vi "App - analyze RUS V6.vi"() -> ()   [LabVIEW 2018] (continued)
{"temperature"=14.948, "lorentzian"={"A (VHz)"=0.0, "f (Hz)"=0.0, "G (Hz)"=0.0, "phi(rad)"=0.0, "Q"=0.0, "Norm  Ampl"=0.0, "bg (V)"=0.0+0.0i, "4corners"={"z (-pi/2)"=0.0+0.0i, "z(inf)"=0.0+0.0i, "z (pi/2)"=0.0+0.0i, "z center"=0.0+0.0i, "z(0)"=0.0+0.0i, "radius"=0.0}}, "timestamp(min)"=2008.2666666656733, "timestamp"=timestamp(3493848317 s since 1904-01-01), "Magn Field(T)"=0.0}, {"temperature"=14.938, "lorentzian"={"A (VHz)"=0.0, "f (Hz)"=0.0, "G (Hz)"=0.0, "phi(rad)"=0.0, "Q"=0.0, "Norm  Ampl"=0.0, "bg (V)"=0.0+0.0i, "4corners"={"z (-pi/2)"=0.0+0.0i, "z(inf)"=0.0+0.0i, "z (pi/2)"=0.0+0.0i, "z center"=0.0+0.0i, "z(0)"=0.0+0.0i, "radius"=0.0}}, "timestamp(min)"=2009.6000000014901, "timestamp"=timestamp(3493848397 s since 1904-01-01), "Magn Field(T)"=0.0}, {"temperature"=14.942, "lorentzian"={"A (VHz)"=0.0, "f (Hz)"=0.0, "G (Hz)"=0.0, "phi(rad)"=0.0, "Q"=0.0, "Norm  Ampl"=0.0, "bg (V)"=0.0+0.0i, "4corners"={"z (-pi/2)"=0.0+0.0i, "z(inf)"=0.0+0.0i, "z (pi/2)"=0.0+0.0i, "z center"=0.0+0.0i, "z(0)"=0.0+0.0i, "radius"=0.0}}, "timestamp(min)"=2010.9166666641831, "timestamp"=timestamp(3493848476 s since 1904-01-01), "Magn Field(T)"=0.0}, {"temperature"=14.929, "lorentzian"={"A (VHz)"=0.0, "f (Hz)"=0.0, "G (Hz)"=0.0, "phi(rad)"=0.0, "Q"=0.0, "Norm  Ampl"=0.0, "bg (V)"=0.0+0.0i, "4corners"={"z (-pi/2)"=0.0+0.0i, "z(inf)"=0.0+0.0i, "z (pi/2)"=0.0+0.0i, "z center"=0.0+0.0i, "z(0)"=0.0+0.0i, "radius"=0.0}}, "timestamp(min)"=2012.2333333343267, "timestamp"=timestamp(3493848555 s since 1904-01-01), "Magn Field(T)"=0.0}, {"temperature"=14.927, "lorentzian"={"A (VHz)"=0.0, "f (Hz)"=0.0, "G (Hz)"=0.0, "phi(rad)"=0.0, "Q"=0.0, "Norm  Ampl"=0.0, "bg (V)"=0.0+0.0i, "4corners"={"z (-pi/2)"=0.0+0.0i, "z(inf)"=0.0+0.0i, "z (pi/2)"=0.0+0.0i, "z center"=0.0+0.0i, "z(0)"=0.0+0.0i, "radius"=0.0}}, "timestamp(min)"=2013.5666666701436, "timestamp"=timestamp(3493848635 s since 1904-01-01), "Magn Field(T)"=0.0}, {"temperature"=14.922, "lorentzian"={"A (VHz)"=0.0, "f (Hz)"=0.0, "G (Hz)"=0.0, "phi(rad)"=0.0, "Q"=0.0, "Norm  Ampl"=0.0, "bg (V)"=0.0+0.0i, "4corners"={"z (-pi/2)"=0.0+0.0i, "z(inf)"=0.0+0.0i, "z (pi/2)"=0.0+0.0i, "z center"=0.0+0.0i, "z(0)"=0.0+0.0i, "radius"=0.0}}, "timestamp(min)"=2014.8833333328366, "timestamp"=timestamp(3493848714 s since 1904-01-01), "Magn Field(T)"=0.0}, {"temperature"=14.929, "lorentzian"={"A (VHz)"=0.0, "f (Hz)"=0.0, "G (Hz)"=0.0, "phi(rad)"=0.0, "Q"=0.0, "Norm  Ampl"=0.0, "bg (V)"=0.0+0.0i, "4corners"={"z (-pi/2)"=0.0+0.0i, "z(inf)"=0.0+0.0i, "z (pi/2)"=0.0+0.0i, "z center"=0.0+0.0i, "z(0)"=0.0+0.0i, "radius"=0.0}}, "timestamp(min)"=2016.2166666686535, "timestamp"=timestamp(3493848794 s since 1904-01-01), "Magn Field(T)"=0.0}, {"temperature"=14.927, "lorentzian"={"A (VHz)"=0.0, "f (Hz)"=0.0, "G (Hz)"=0.0, "phi(rad)"=0.0, "Q"=0.0, "Norm  Ampl"=0.0, "bg (V)"=0.0+0.0i, "4corners"={"z (-pi/2)"=0.0+0.0i, "z(inf)"=0.0+0.0i, "z (pi/2)"=0.0+0.0i, "z center"=0.0+0.0i, "z(0)"=0.0+0.0i, "radius"=0.0}}, "timestamp(min)"=2017.5333333313465, "timestamp"=timestamp(3493848873 s since 1904-01-01), "Magn Field(T)"=0.0}, {"temperature"=14.926, "lorentzian"={"A (VHz)"=0.0, "f (Hz)"=0.0, "G (Hz)"=0.0, "phi(rad)"=0.0, "Q"=0.0, "Norm  Ampl"=0.0, "bg (V)"=0.0+0.0i, "4corners"={"z (-pi/2)"=0.0+0.0i, "z(inf)"=0.0+0.0i, "z (pi/2)"=0.0+0.0i, "z center"=0.0+0.0i, "z(0)"=0.0+0.0i, "radius"=0.0}}, "timestamp(min)"=2018.8500000014901, "timestamp"=timestamp(3493848952 s since 1904-01-01), "Magn Field(T)"=0.0}, {"temperature"=14.912, "lorentzian"={"A (VHz)"=0.0, "f (Hz)"=0.0, "G (Hz)"=0.0, "phi(rad)"=0.0, "Q"=0.0, "Norm  Ampl"=0.0, "bg (V)"=0.0+0.0i, "4corners"={"z (-pi/2)"=0.0+0.0i, "z(inf)"=0.0+0.0i, "z (pi/2)"=0.0+0.0i, "z center"=0.0+0.0i, "z(0)"=0.0+0.0i, "radius"=0.0}}, "timestamp(min)"=2020.183333337307, "timestamp"=timestamp(3493849032 s since 1904-01-01), "Magn Field(T)"=0.0}, {"temperature"=14.915, "lorentzian"={"A (VHz)"=0.0, "f (Hz)"=0.0, "G (Hz)"=0.0, "phi(rad)"=0.0, "Q"=0.0, "Norm  Ampl"=0.0, "bg (V)"=0.0+0.0i, "4corners"={"z (-pi/2)"=0.0+0.0i, "z(inf)"=0.0+0.0i, "z (pi/2)"=0.0+0.0i, "z center"=0.0+0.0i, "z(0)"=0.0+0.0i, "radius"=0.0}}, "timestamp(min)"=2021.5, "timestamp"=timestamp(3493849111 s since 1904-01-01), "Magn Field(T)"=0.0}, {"temperature"=14.912, "lorentzian"={"A (VHz)"=0.0, "f (Hz)"=0.0, "G (Hz)"=0.0, "phi(rad)"=0.0, "Q"=0.0, "Norm  Ampl"=0.0, "bg (V)"=0.0+0.0i, "4corners"={"z (-pi/2)"=0.0+0.0i, "z(inf)"=0.0+0.0i, "z (pi/2)"=0.0+0.0i, "z center"=0.0+0.0i, "z(0)"=0.0+0.0i, "radius"=0.0}}, "timestamp(min)"=2022.8166666701436, "timestamp"=timestamp(3493849190 s since 1904-01-01), "Magn Field(T)"=0.0}, {"temperature"=14.91, "lorentzian"={"A (VHz)"=0.0, "f (Hz)"=0.0, "G (Hz)"=0.0, "phi(rad)"=0.0, "Q"=0.0, "Norm  Ampl"=0.0, "bg (V)"=0.0+0.0i, "4corners"={"z (-pi/2)"=0.0+0.0i, "z(inf)"=0.0+0.0i, "z (pi/2)"=0.0+0.0i, "z center"=0.0+0.0i, "z(0)"=0.0+0.0i, "radius"=0.0}}, "timestamp(min)"=2024.1499999985099, "timestamp"=timestamp(3493849270 s since 1904-01-01), "Magn Field(T)"=0.0}, {"temperature"=14.907, "lorentzian"={"A (VHz)"=0.0, "f (Hz)"=0.0, "G (Hz)"=0.0, "phi(rad)"=0.0, "Q"=0.0, "Norm  Ampl"=0.0, "bg (V)"=0.0+0.0i, "4corners"={"z (-pi/2)"=0.0+0.0i, "z(inf)"=0.0+0.0i, "z (pi/2)"=0.0+0.0i, "z center"=0.0+0.0i, "z(0)"=0.0+0.0i, "radius"=0.0}}, "timestamp(min)"=2025.4666666686535, "timestamp"=timestamp(3493849349 s since 1904-01-01), "Magn Field(T)"=0.0}, {"temperature"=14.908, "lorentzian"={"A (VHz)"=0.0, "f (Hz)"=0.0, "G (Hz)"=0.0, "phi(rad)"=0.0, "Q"=0.0, "Norm  Ampl"=0.0, "bg (V)"=0.0+0.0i, "4corners"={"z (-pi/2)"=0.0+0.0i, "z(inf)"=0.0+0.0i, "z (pi/2)"=0.0+0.0i, "z center"=0.0+0.0i, "z(0)"=0.0+0.0i, "radius"=0.0}}, "timestamp(min)"=2026.8000000044703, "timestamp"=timestamp(3493849429 s since 1904-01-01), "Magn Field(T)"=0.0}, {"temperature"=14.9, "lorentzian"={"A (VHz)"=0.0, "f (Hz)"=0.0, "G (Hz)"=0.0, "phi(rad)"=0.0, "Q"=0.0, "Norm  Ampl"=0.0, "bg (V)"=0.0+0.0i, "4corners"={"z (-pi/2)"=0.0+0.0i, "z(inf)"=0.0+0.0i, "z (pi/2)"=0.0+0.0i, "z center"=0.0+0.0i, "z(0)"=0.0+0.0i, "radius"=0.0}}, "timestamp(min)"=2028.1166666671634, "timestamp"=timestamp(3493849508 s since 1904-01-01), "Magn Field(T)"=0.0}, {"temperature"=14.9, "lorentzian"={"A (VHz)"=0.0, "f (Hz)"=0.0, "G (Hz)"=0.0, "phi(rad)"=0.0, "Q"=0.0, "Norm  Ampl"=0.0, "bg (V)"=0.0+0.0i, "4corners"={"z (-pi/2)"=0.0+0.0i, "z(inf)"=0.0+0.0i, "z (pi/2)"=0.0+0.0i, "z center"=0.0+0.0i, "z(0)"=0.0+0.0i, "radius"=0.0}}, "timestamp(min)"=2029.433333337307, "timestamp"=timestamp(3493849587 s since 1904-01-01), "Magn Field(T)"=0.0}, {"temperature"=14.895, "lorentzian"={"A (VHz)"=0.0, "f (Hz)"=0.0, "G (Hz)"=0.0, "phi(rad)"=0.0, "Q"=0.0, "Norm  Ampl"=0.0, "bg (V)"=0.0+0.0i, "4corners"={"z (-pi/2)"=0.0+0.0i, "z(inf)"=0.0+0.0i, "z (pi/2)"=0.0+0.0i, "z center"=0.0+0.0i, "z(0)"=0.0+0.0i, "radius"=0.0}}, "timestamp(min)"=2030.7666666656733, "timestamp"=timestamp(3493849667 s since 1904-01-01), "Magn Field(T)"=0.0}, {"temperature"=14.89, "lorentzian"={"A (VHz)"=0.0, "f (Hz)"=0.0, "G (Hz)"=0.0, "phi(rad)"=0.0, "Q"=0.0, "Norm  Ampl"=0.0, "bg (V)"=0.0+0.0i, "4corners"={"z (-pi/2)"=0.0+0.0i, "z(inf)"=0.0+0.0i, "z (pi/2)"=0.0+0.0i, "z center"=0.0+0.0i, "z(0)"=0.0+0.0i, "radius"=0.0}}, "timestamp(min)"=2032.0833333358169, "timestamp"=timestamp(3493849746 s since 1904-01-01), "Magn Field(T)"=0.0}, {"temperature"=14.886, "lorentzian"={"A (VHz)"=0.0, "f (Hz)"=0.0, "G (Hz)"=0.0, "phi(rad)"=0.0, "Q"=0.0, "Norm  Ampl"=0.0, "bg (V)"=0.0+0.0i, "4corners"={"z (-pi/2)"=0.0+0.0i, "z(inf)"=0.0+0.0i, "z (pi/2)"=0.0+0.0i, "z center"=0.0+0.0i, "z(0)"=0.0+0.0i, "radius"=0.0}}, "timestamp(min)"=2033.4166666641831, "timestamp"=timestamp(3493849826 s since 1904-01-01), "Magn Field(T)"=0.0}, {"temperature"=14.883, "lorentzian"={"A (VHz)"=0.0, "f (Hz)"=0.0, "G (Hz)"=0.0, "phi(rad)"=0.0, "Q"=0.0, "Norm  Ampl"=0.0, "bg (V)"=0.0+0.0i, "4corners"={"z (-pi/2)"=0.0+0.0i, "z(inf)"=0.0+0.0i, "z (pi/2)"=0.0+0.0i, "z center"=0.0+0.0i, "z(0)"=0.0+0.0i, "radius"=0.0}}, "timestamp(min)"=2034.7333333343267, "timestamp"=timestamp(3493849905 s since 1904-01-01), "Magn Field(T)"=0.0}, {"temperature"=14.876, "lorentzian"={"A (VHz)"=0.0, "f (Hz)"=0.0, "G (Hz)"=0.0, "phi(rad)"=0.0, "Q"=0.0, "Norm  Ampl"=0.0, "bg (V)"=0.0+0.0i, "4corners"={"z (-pi/2)"=0.0+0.0i, "z(inf)"=0.0+0.0i, "z (pi/2)"=0.0+0.0i, "z center"=0.0+0.0i, "z(0)"=0.0+0.0i, "radius"=0.0}}, "timestamp(min)"=2036.0500000044703, "timestamp"=timestamp(3493849984 s since 1904-01-01), "Magn Field(T)"=0.0}, {"temperature"=14.875, "lorentzian"={"A (VHz)"=0.0, "f (Hz)"=0.0, "G (Hz)"=0.0, "phi(rad)"=0.0, "Q"=0.0, "Norm  Ampl"=0.0, "bg (V)"=0.0+0.0i, "4corners"={"z (-pi/2)"=0.0+0.0i, "z(inf)"=0.0+0.0i, "z (pi/2)"=0.0+0.0i, "z center"=0.0+0.0i, "z(0)"=0.0+0.0i, "radius"=0.0}}, "timestamp(min)"=2037.3833333328366, "timestamp"=timestamp(3493850064 s since 1904-01-01), "Magn Field(T)"=0.0}, {"temperature"=14.872, "lorentzian"={"A (VHz)"=0.0, "f (Hz)"=0.0, "G (Hz)"=0.0, "phi(rad)"=0.0, "Q"=0.0, "Norm  Ampl"=0.0, "bg (V)"=0.0+0.0i, "4corners"={"z (-pi/2)"=0.0+0.0i, "z(inf)"=0.0+0.0i, "z (pi/2)"=0.0+0.0i, "z center"=0.0+0.0i, "z(0)"=0.0+0.0i, "radius"=0.0}}, "timestamp(min)"=2038.7000000029802, "timestamp"=timestamp(3493850143 s since 1904-01-01), "Magn Field(T)"=0.0}, {"temperature"=14.874, "lorentzian"={"A (VHz)"=0.0, "f (Hz)"=0.0, "G (Hz)"=0.0, "phi(rad)"=0.0, "Q"=0.0, "Norm  Ampl"=0.0, "bg (V)"=0.0+0.0i, "4corners"={"z (-pi/2)"=0.0+0.0i, "z(inf)"=0.0+0.0i, "z (pi/2)"=0.0+0.0i, "z center"=0.0+0.0i, "z(0)"=0.0+0.0i, "radius"=0.0}}, "timestamp(min)"=2040.0166666656733, "timestamp"=timestamp(3493850222 s since 1904-01-01), "Magn Field(T)"=0.0}, {"temperature"=14.877, "lorentzian"={"A (VHz)"=0.0, "f (Hz)"=0.0, "G (Hz)"=0.0, "phi(rad)"=0.0, "Q"=0.0, "Norm  Ampl"=0.0, "bg (V)"=0.0+0.0i, "4corners"={"z (-pi/2)"=0.0+0.0i, "z(inf)"=0.0+0.0i, "z (pi/2)"=0.0+0.0i, "z center"=0.0+0.0i, "z(0)"=0.0+0.0i, "radius"=0.0}}, "timestamp(min)"=2041.3500000014901, "timestamp"=timestamp(3493850302 s since 1904-01-01), "Magn Field(T)"=0.0}, {"temperature"=14.872, "lorentzian"={"A (VHz)"=0.0, "f (Hz)"=0.0, "G (Hz)"=0.0, "phi(rad)"=0.0, "Q"=0.0, "Norm  Ampl"=0.0, "bg (V)"=0.0+0.0i, "4corners"={"z (-pi/2)"=0.0+0.0i, "z(inf)"=0.0+0.0i, "z (pi/2)"=0.0+0.0i, "z center"=0.0+0.0i, "z(0)"=0.0+0.0i, "radius"=0.0}}, "timestamp(min)"=2042.6666666641831, "timestamp"=timestamp(3493850381 s since 1904-01-01), "Magn Field(T)"=0.0}, {"temperature"=14.873, "lorentzian"={"A (VHz)"=0.0, "f (Hz)"=0.0, "G (Hz)"=0.0, "phi(rad)"=0.0, "Q"=0.0, "Norm  Ampl"=0.0, "bg (V)"=0.0+0.0i, "4corners"={"z (-pi/2)"=0.0+0.0i, "z(inf)"=0.0+0.0i, "z (pi/2)"=0.0+0.0i, "z center"=0.0+0.0i, "z(0)"=0.0+0.0i, "radius"=0.0}}, "timestamp(min)"=2044.0, "timestamp"=timestamp(3493850461 s since 1904-01-01), "Magn Field(T)"=0.0}, {"temperature"=14.873, "lorentzian"={"A (VHz)"=0.0, "f (Hz)"=0.0, "G (Hz)"=0.0, "phi(rad)"=0.0, "Q"=0.0, "Norm  Ampl"=0.0, "bg (V)"=0.0+0.0i, "4corners"={"z (-pi/2)"=0.0+0.0i, "z(inf)"=0.0+0.0i, "z (pi/2)"=0.0+0.0i, "z center"=0.0+0.0i, "z(0)"=0.0+0.0i, "radius"=0.0}}, "timestamp(min)"=2045.3166666701436, "timestamp"=timestamp(3493850540 s since 1904-01-01), "Magn Field(T)"=0.0}, {"temperature"=14.868, "lorentzian"={"A (VHz)"=0.0, "f (Hz)"=0.0, "G (Hz)"=0.0, "phi(rad)"=0.0, "Q"=0.0, "Norm  Ampl"=0.0, "bg (V)"=0.0+0.0i, "4corners"={"z (-pi/2)"=0.0+0.0i, "z(inf)"=0.0+0.0i, "z (pi/2)"=0.0+0.0i, "z center"=0.0+0.0i, "z(0)"=0.0+0.0i, "radius"=0.0}}, "timestamp(min)"=2046.6333333328366, "timestamp"=timestamp(3493850619 s since 1904-01-01), "Magn Field(T)"=0.0}, {"temperature"=14.859, "lorentzian"={"A (VHz)"=0.0, "f (Hz)"=0.0, "G (Hz)"=0.0, "phi(rad)"=0.0, "Q"=0.0, "Norm  Ampl"=0.0, "bg (V)"=0.0+0.0i, "4corners"={"z (-pi/2)"=0.0+0.0i, "z(inf)"=0.0+0.0i, "z (pi/2)"=0.0+0.0i, "z center"=0.0+0.0i, "z(0)"=0.0+0.0i, "radius"=0.0}}, "timestamp(min)"=2047.9666666686535, "timestamp"=timestamp(3493850699 s since 1904-01-01), "Magn Field(T)"=0.0}, {"temperature"=14.866, "lorentzian"={"A (VHz)"=0.0, "f (Hz)"=0.0, "G (Hz)"=0.0, "phi(rad)"=0.0, "Q"=0.0, "Norm  Ampl"=0.0, "bg (V)"=0.0+0.0i, "4corners"={"z (-pi/2)"=0.0+0.0i, "z(inf)"=0.0+0.0i, "z (pi/2)"=0.0+0.0i, "z center"=0.0+0.0i, "z(0)"=0.0+0.0i, "radius"=0.0}}, "timestamp(min)"=2049.2833333313465, "timestamp"=timestamp(3493850778 s since 1904-01-01), "Magn Field(T)"=0.0}, {"temperature"=14.858, "lorentzian"={"A (VHz)"=0.0, "f (Hz)"=0.0, "G (Hz)"=0.0, "phi(rad)"=0.0, "Q"=0.0, "Norm  Ampl"=0.0, "bg (V)"=0.0+0.0i, "4corners"={"z (-pi/2)"=0.0+0.0i, "z(inf)"=0.0+0.0i, "z (pi/2)"=0.0+0.0i, "z center"=0.0+0.0i, "z(0)"=0.0+0.0i, "radius"=0.0}}, "timestamp(min)"=2050.60000000149, "timestamp"=timestamp(3493850857 s since 1904-01-01), "Magn Field(T)"=0.0}, {"temperature"=14.86, "lorentzian"={"A (VHz)"=0.0, "f (Hz)"=0.0, "G (Hz)"=0.0, "phi(rad)"=0.0, "Q"=0.0, "Norm  Ampl"=0.0, "bg (V)"=0.0+0.0i, "4corners"={"z (-pi/2)"=0.0+0.0i, "z(inf)"=0.0+0.0i, "z (pi/2)"=0.0+0.0i, "z center"=0.0+0.0i, "z(0)"=0.0+0.0i, "radius"=0.0}}, "timestamp(min)"=2051.933333337307, "timestamp"=timestamp(3493850937 s since 1904-01-01), "Magn Field(T)"=0.0}, {"temperature"=14.866, "lorentzian"={"A (VHz)"=0.0, "f (Hz)"=0.0, "G (Hz)"=0.0, "phi(rad)"=0.0, "Q"=0.0, "Norm  Ampl"=0.0, "bg (V)"=0.0+0.0i, "4corners"={"z (-pi/2)"=0.0+0.0i, "z(inf)"=0.0+0.0i, "z (pi/2)"=0.0+0.0i, "z center"=0.0+0.0i, "z(0)"=0.0+0.0i, "radius"=0.0}}, "timestamp(min)"=2053.25, "timestamp"=timestamp(3493851016 s since 1904-01-01), "Magn Field(T)"=0.0}, {"temperature"=14.857, "lorentzian"={"A (VHz)"=0.0, "f (Hz)"=0.0, "G (Hz)"=0.0, "phi(rad)"=0.0, "Q"=0.0, "Norm  Ampl"=0.0, "bg (V)"=0.0+0.0i, "4corners"={"z (-pi/2)"=0.0+0.0i, "z(inf)"=0.0+0.0i, "z (pi/2)"=0.0+0.0i, "z center"=0.0+0.0i, "z(0)"=0.0+0.0i, "radius"=0.0}}, "timestamp(min)"=2054.583333335817, "timestamp"=timestamp(3493851096 s since 1904-01-01), "Magn Field(T)"=0.0}, {"temperature"=14.853, "lorentzian"={"A (VHz)"=0.0, "f (Hz)"=0.0, "G (Hz)"=0.0, "phi(rad)"=0.0, "Q"=0.0, "Norm  Ampl"=0.0, "bg (V)"=0.0+0.0i, "4corners"={"z (-pi/2)"=0.0+0.0i, "z(inf)"=0.0+0.0i, "z (pi/2)"=0.0+0.0i, "z center"=0.0+0.0i, "z(0)"=0.0+0.0i, "radius"=0.0}}, "timestamp(min)"=2055.89999999851, "timestamp"=timestamp(3493851175 s since 1904-01-01), "Magn Field(T)"=0.0}, {"temperature"=14.852, "lorentzian"={"A (VHz)"=0.0, "f (Hz)"=0.0, "G (Hz)"=0.0, "phi(rad)"=0.0, "Q"=0.0, "Norm  Ampl"=0.0, "bg (V)"=0.0+0.0i, "4corners"={"z (-pi/2)"=0.0+0.0i, "z(inf)"=0.0+0.0i, "z (pi/2)"=0.0+0.0i, "z center"=0.0+0.0i, "z(0)"=0.0+0.0i, "radius"=0.0}}, "timestamp(min)"=2057.2166666686535, "timestamp"=timestamp(3493851254 s since 1904-01-01), "Magn Field(T)"=0.0}, {"temperature"=14.844, "lorentzian"={"A (VHz)"=0.0, "f (Hz)"=0.0, "G (Hz)"=0.0, "phi(rad)"=0.0, "Q"=0.0, "Norm  Ampl"=0.0, "bg (V)"=0.0+0.0i, "4corners"={"z (-pi/2)"=0.0+0.0i, "z(inf)"=0.0+0.0i, "z (pi/2)"=0.0+0.0i, "z center"=0.0+0.0i, "z(0)"=0.0+0.0i, "radius"=0.0}}, "timestamp(min)"=2058.5500000044703, "timestamp"=timestamp(3493851334 s since 1904-01-01), "Magn Field(T)"=0.0}, {"temperature"=14.841, "lorentzian"={"A (VHz)"=0.0, "f (Hz)"=0.0, "G (Hz)"=0.0, "phi(rad)"=0.0, "Q"=0.0, "Norm  Ampl"=0.0, "bg (V)"=0.0+0.0i, "4corners"={"z (-pi/2)"=0.0+0.0i, "z(inf)"=0.0+0.0i, "z (pi/2)"=0.0+0.0i, "z center"=0.0+0.0i, "z(0)"=0.0+0.0i, "radius"=0.0}}, "timestamp(min)"=2059.8666666671634, "timestamp"=timestamp(3493851413 s since 1904-01-01), "Magn Field(T)"=0.0}, {"temperature"=14.835, "lorentzian"={"A (VHz)"=0.0, "f (Hz)"=0.0, "G (Hz)"=0.0, "phi(rad)"=0.0, "Q"=0.0, "Norm  Ampl"=0.0, "bg (V)"=0.0+0.0i, "4corners"={"z (-pi/2)"=0.0+0.0i, "z(inf)"=0.0+0.0i, "z (pi/2)"=0.0+0.0i, "z center"=0.0+0.0i, "z(0)"=0.0+0.0i, "radius"=0.0}}, "timestamp(min)"=2061.183333337307, "timestamp"=timestamp(3493851492 s since 1904-01-01), "Magn Field(T)"=0.0}, {"temperature"=14.822, "lorentzian"={"A (VHz)"=0.0, "f (Hz)"=0.0, "G (Hz)"=0.0, "phi(rad)"=0.0, "Q"=0.0, "Norm  Ampl"=0.0, "bg (V)"=0.0+0.0i, "4corners"={"z (-pi/2)"=0.0+0.0i, "z(inf)"=0.0+0.0i, "z (pi/2)"=0.0+0.0i, "z center"=0.0+0.0i, "z(0)"=0.0+0.0i, "radius"=0.0}}, "timestamp(min)"=2062.5166666656733, "timestamp"=timestamp(3493851572 s since 1904-01-01), "Magn Field(T)"=0.0}, {"temperature"=14.821, "lorentzian"={"A (VHz)"=0.0, "f (Hz)"=0.0, "G (Hz)"=0.0, "phi(rad)"=0.0, "Q"=0.0, "Norm  Ampl"=0.0, "bg (V)"=0.0+0.0i, "4corners"={"z (-pi/2)"=0.0+0.0i, "z(inf)"=0.0+0.0i, "z (pi/2)"=0.0+0.0i, "z center"=0.0+0.0i, "z(0)"=0.0+0.0i, "radius"=0.0}}, "timestamp(min)"=2063.833333335817, "timestamp"=timestamp(3493851651 s since 1904-01-01), "Magn Field(T)"=0.0}, {"temperature"=14.824, "lorentzian"={"A (VHz)"=0.0, "f (Hz)"=0.0, "G (Hz)"=0.0, "phi(rad)"=0.0, "Q"=0.0, "Norm  Ampl"=0.0, "bg (V)"=0.0+0.0i, "4corners"={"z (-pi/2)"=0.0+0.0i, "z(inf)"=0.0+0.0i, "z (pi/2)"=0.0+0.0i, "z center"=0.0+0.0i, "z(0)"=0.0+0.0i, "radius"=0.0}}, "timestamp(min)"=2065.166666664183, "timestamp"=timestamp(3493851731 s since 1904-01-01), "Magn Field(T)"=0.0}, {"temperature"=14.817, "lorentzian"={"A (VHz)"=0.0, "f (Hz)"=0.0, "G (Hz)"=0.0, "phi(rad)"=0.0, "Q"=0.0, "Norm  Ampl"=0.0, "bg (V)"=0.0+0.0i, "4corners"={"z (-pi/2)"=0.0+0.0i, "z(inf)"=0.0+0.0i, "z (pi/2)"=0.0+0.0i, "z center"=0.0+0.0i, "z(0)"=0.0+0.0i, "radius"=0.0}}, "timestamp(min)"=2066.4833333343267, "timestamp"=timestamp(3493851810 s since 1904-01-01), "Magn Field(T)"=0.0}, {"temperature"=14.811, "lorentzian"={"A (VHz)"=0.0, "f (Hz)"=0.0, "G (Hz)"=0.0, "phi(rad)"=0.0, "Q"=0.0, "Norm  Ampl"=0.0, "bg (V)"=0.0+0.0i, "4corners"={"z (-pi/2)"=0.0+0.0i, "z(inf)"=0.0+0.0i, "z (pi/2)"=0.0+0.0i, "z center"=0.0+0.0i, "z(0)"=0.0+0.0i, "radius"=0.0}}, "timestamp(min)"=2067.8000000044703, "timestamp"=timestamp(3493851889 s since 1904-01-01), "Magn Field(T)"=0.0}, {"temperature"=14.805, "lorentzian"={"A (VHz)"=0.0, "f (Hz)"=0.0, "G (Hz)"=0.0, "phi(rad)"=0.0, "Q"=0.0, "Norm  Ampl"=0.0, "bg (V)"=0.0+0.0i, "4corners"={"z (-pi/2)"=0.0+0.0i, "z(inf)"=0.0+0.0i, "z (pi/2)"=0.0+0.0i, "z center"=0.0+0.0i, "z(0)"=0.0+0.0i, "radius"=0.0}}, "timestamp(min)"=2069.1333333328366, "timestamp"=timestamp(3493851969 s since 1904-01-01), "Magn Field(T)"=0.0}, {"temperature"=14.791, "lorentzian"={"A (VHz)"=0.0, "f (Hz)"=0.0, "G (Hz)"=0.0, "phi(rad)"=0.0, "Q"=0.0, "Norm  Ampl"=0.0, "bg (V)"=0.0+0.0i, "4corners"={"z (-pi/2)"=0.0+0.0i, "z(inf)"=0.0+0.0i, "z (pi/2)"=0.0+0.0i, "z center"=0.0+0.0i, "z(0)"=0.0+0.0i, "radius"=0.0}}, "timestamp(min)"=2070.4500000029802, "timestamp"=timestamp(3493852048 s since 1904-01-01), "Magn Field(T)"=0.0}, {"temperature"=14.787, "lorentzian"={"A (VHz)"=0.0, "f (Hz)"=0.0, "G (Hz)"=0.0, "phi(rad)"=0.0, "Q"=0.0, "Norm  Ampl"=0.0, "bg (V)"=0.0+0.0i, "4corners"={"z (-pi/2)"=0.0+0.0i, "z(inf)"=0.0+0.0i, "z (pi/2)"=0.0+0.0i, "z center"=0.0+0.0i, "z(0)"=0.0+0.0i, "radius"=0.0}}, "timestamp(min)"=2071.7833333313465, "timestamp"=timestamp(3493852128 s since 1904-01-01), "Magn Field(T)"=0.0}, {"temperature"=14.778, "lorentzian"={"A (VHz)"=0.0, "f (Hz)"=0.0, "G (Hz)"=0.0, "phi(rad)"=0.0, "Q"=0.0, "Norm  Ampl"=0.0, "bg (V)"=0.0+0.0i, "4corners"={"z (-pi/2)"=0.0+0.0i, "z(inf)"=0.0+0.0i, "z (pi/2)"=0.0+0.0i, "z center"=0.0+0.0i, "z(0)"=0.0+0.0i, "radius"=0.0}}, "timestamp(min)"=2073.10000000149, "timestamp"=timestamp(3493852207 s since 1904-01-01), "Magn Field(T)"=0.0}, {"temperature"=14.773, "lorentzian"={"A (VHz)"=0.0, "f (Hz)"=0.0, "G (Hz)"=0.0, "phi(rad)"=0.0, "Q"=0.0, "Norm  Ampl"=0.0, "bg (V)"=0.0+0.0i, "4corners"={"z (-pi/2)"=0.0+0.0i, "z(inf)"=0.0+0.0i, "z (pi/2)"=0.0+0.0i, "z center"=0.0+0.0i, "z(0)"=0.0+0.0i, "radius"=0.0}}, "timestamp(min)"=2074.416666664183, "timestamp"=timestamp(3493852286 s since 1904-01-01), "Magn Field(T)"=0.0}, {"temperature"=14.769, "lorentzian"={"A (VHz)"=0.0, "f (Hz)"=0.0, "G (Hz)"=0.0, "phi(rad)"=0.0, "Q"=0.0, "Norm  Ampl"=0.0, "bg (V)"=0.0+0.0i, "4corners"={"z (-pi/2)"=0.0+0.0i, "z(inf)"=0.0+0.0i, "z (pi/2)"=0.0+0.0i, "z center"=0.0+0.0i, "z(0)"=0.0+0.0i, "radius"=0.0}}, "timestamp(min)"=2075.75, "timestamp"=timestamp(3493852366 s since 1904-01-01), "Magn Field(T)"=0.0}, {"temperature"=14.763, "lorentzian"={"A (VHz)"=0.0, "f (Hz)"=0.0, "G (Hz)"=0.0, "phi(rad)"=0.0, "Q"=0.0, "Norm  Ampl"=0.0, "bg (V)"=0.0+0.0i, "4corners"={"z (-pi/2)"=0.0+0.0i, "z(inf)"=0.0+0.0i, "z (pi/2)"=0.0+0.0i, "z center"=0.0+0.0i, "z(0)"=0.0+0.0i, "radius"=0.0}}, "timestamp(min)"=2077.0666666701436, "timestamp"=timestamp(3493852445 s since 1904-01-01), "Magn Field(T)"=0.0}, {"temperature"=14.753, "lorentzian"={"A (VHz)"=0.0, "f (Hz)"=0.0, "G (Hz)"=0.0, "phi(rad)"=0.0, "Q"=0.0, "Norm  Ampl"=0.0, "bg (V)"=0.0+0.0i, "4corners"={"z (-pi/2)"=0.0+0.0i, "z(inf)"=0.0+0.0i, "z (pi/2)"=0.0+0.0i, "z center"=0.0+0.0i, "z(0)"=0.0+0.0i, "radius"=0.0}}, "timestamp(min)"=2078.3833333328366, "timestamp"=timestamp(3493852524 s since 1904-01-01), "Magn Field(T)"=0.0}, {"temperature"=14.749, "lorentzian"={"A (VHz)"=0.0, "f (Hz)"=0.0, "G (Hz)"=0.0, "phi(rad)"=0.0, "Q"=0.0, "Norm  Ampl"=0.0, "bg (V)"=0.0+0.0i, "4corners"={"z (-pi/2)"=0.0+0.0i, "z(inf)"=0.0+0.0i, "z (pi/2)"=0.0+0.0i, "z center"=0.0+0.0i, "z(0)"=0.0+0.0i, "radius"=0.0}}, "timestamp(min)"=2079.7166666686535, "timestamp"=timestamp(3493852604 s since 1904-01-01), "Magn Field(T)"=0.0}, {"temperature"=14.747, "lorentzian"={"A (VHz)"=0.0, "f (Hz)"=0.0, "G (Hz)"=0.0, "phi(rad)"=0.0, "Q"=0.0, "Norm  Ampl"=0.0, "bg (V)"=0.0+0.0i, "4corners"={"z (-pi/2)"=0.0+0.0i, "z(inf)"=0.0+0.0i, "z (pi/2)"=0.0+0.0i, "z center"=0.0+0.0i, "z(0)"=0.0+0.0i, "radius"=0.0}}, "timestamp(min)"=2081.0333333313465, "timestamp"=timestamp(3493852683 s since 1904-01-01), "Magn Field(T)"=0.0}, {"temperature"=14.742, "lorentzian"={"A (VHz)"=0.0, "f (Hz)"=0.0, "G (Hz)"=0.0, "phi(rad)"=0.0, "Q"=0.0, "Norm  Ampl"=0.0, "bg (V)"=0.0+0.0i, "4corners"={"z (-pi/2)"=0.0+0.0i, "z(inf)"=0.0+0.0i, "z (pi/2)"=0.0+0.0i, "z center"=0.0+0.0i, "z(0)"=0.0+0.0i, "radius"=0.0}}, "timestamp(min)"=2082.3666666671634, "timestamp"=timestamp(3493852763 s since 1904-01-01), "Magn Field(T)"=0.0}, {"temperature"=14.739, "lorentzian"={"A (VHz)"=0.0, "f (Hz)"=0.0, "G (Hz)"=0.0, "phi(rad)"=0.0, "Q"=0.0, "Norm  Ampl"=0.0, "bg (V)"=0.0+0.0i, "4corners"={"z (-pi/2)"=0.0+0.0i, "z(inf)"=0.0+0.0i, "z (pi/2)"=0.0+0.0i, "z center"=0.0+0.0i, "z(0)"=0.0+0.0i, "radius"=0.0}}, "timestamp(min)"=2083.683333337307, "timestamp"=timestamp(3493852842 s since 1904-01-01), "Magn Field(T)"=0.0}, {"temperature"=14.735, "lorentzian"={"A (VHz)"=0.0, "f (Hz)"=0.0, "G (Hz)"=0.0, "phi(rad)"=0.0, "Q"=0.0, "Norm  Ampl"=0.0, "bg (V)"=0.0+0.0i, "4corners"={"z (-pi/2)"=0.0+0.0i, "z(inf)"=0.0+0.0i, "z (pi/2)"=0.0+0.0i, "z center"=0.0+0.0i, "z(0)"=0.0+0.0i, "radius"=0.0}}, "timestamp(min)"=2085.0, "timestamp"=timestamp(3493852921 s since 1904-01-01), "Magn Field(T)"=0.0}, {"temperature"=14.73, "lorentzian"={"A (VHz)"=0.0, "f (Hz)"=0.0, "G (Hz)"=0.0, "phi(rad)"=0.0, "Q"=0.0, "Norm  Ampl"=0.0, "bg (V)"=0.0+0.0i, "4corners"={"z (-pi/2)"=0.0+0.0i, "z(inf)"=0.0+0.0i, "z (pi/2)"=0.0+0.0i, "z center"=0.0+0.0i, "z(0)"=0.0+0.0i, "radius"=0.0}}, "timestamp(min)"=2086.333333335817, "timestamp"=timestamp(3493853001 s since 1904-01-01), "Magn Field(T)"=0.0}, {"temperature"=14.731, "lorentzian"={"A (VHz)"=0.0, "f (Hz)"=0.0, "G (Hz)"=0.0, "phi(rad)"=0.0, "Q"=0.0, "Norm  Ampl"=0.0, "bg (V)"=0.0+0.0i, "4corners"={"z (-pi/2)"=0.0+0.0i, "z(inf)"=0.0+0.0i, "z (pi/2)"=0.0+0.0i, "z center"=0.0+0.0i, "z(0)"=0.0+0.0i, "radius"=0.0}}, "timestamp(min)"=2087.64999999851, "timestamp"=timestamp(3493853080 s since 1904-01-01), "Magn Field(T)"=0.0}, {"temperature"=14.74, "lorentzian"={"A (VHz)"=0.0, "f (Hz)"=0.0, "G (Hz)"=0.0, "phi(rad)"=0.0, "Q"=0.0, "Norm  Ampl"=0.0, "bg (V)"=0.0+0.0i, "4corners"={"z (-pi/2)"=0.0+0.0i, "z(inf)"=0.0+0.0i, "z (pi/2)"=0.0+0.0i, "z center"=0.0+0.0i, "z(0)"=0.0+0.0i, "radius"=0.0}}, "timestamp(min)"=2088.9666666686535, "timestamp"=timestamp(3493853159 s since 1904-01-01), "Magn Field(T)"=0.0}, {"temperature"=14.735, "lorentzian"={"A (VHz)"=0.0, "f (Hz)"=0.0, "G (Hz)"=0.0, "phi(rad)"=0.0, "Q"=0.0, "Norm  Ampl"=0.0, "bg (V)"=0.0+0.0i, "4corners"={"z (-pi/2)"=0.0+0.0i, "z(inf)"=0.0+0.0i, "z (pi/2)"=0.0+0.0i, "z center"=0.0+0.0i, "z(0)"=0.0+0.0i, "radius"=0.0}}, "timestamp(min)"=2090.3000000044703, "timestamp"=timestamp(3493853239 s since 1904-01-01), "Magn Field(T)"=0.0}, {"temperature"=14.742, "lorentzian"={"A (VHz)"=0.0, "f (Hz)"=0.0, "G (Hz)"=0.0, "phi(rad)"=0.0, "Q"=0.0, "Norm  Ampl"=0.0, "bg (V)"=0.0+0.0i, "4corners"={"z (-pi/2)"=0.0+0.0i, "z(inf)"=0.0+0.0i, "z (pi/2)"=0.0+0.0i, "z center"=0.0+0.0i, "z(0)"=0.0+0.0i, "radius"=0.0}}, "timestamp(min)"=2091.6166666671634, "timestamp"=timestamp(3493853318 s since 1904-01-01), "Magn Field(T)"=0.0}, {"temperature"=14.735, "lorentzian"={"A (VHz)"=0.0, "f (Hz)"=0.0, "G (Hz)"=0.0, "phi(rad)"=0.0, "Q"=0.0, "Norm  Ampl"=0.0, "bg (V)"=0.0+0.0i, "4corners"={"z (-pi/2)"=0.0+0.0i, "z(inf)"=0.0+0.0i, "z (pi/2)"=0.0+0.0i, "z center"=0.0+0.0i, "z(0)"=0.0+0.0i, "radius"=0.0}}, "timestamp(min)"=2092.9500000029802, "timestamp"=timestamp(3493853398 s since 1904-01-01), "Magn Field(T)"=0.0}, {"temperature"=14.732, "lorentzian"={"A (VHz)"=0.0, "f (Hz)"=0.0, "G (Hz)"=0.0, "phi(rad)"=0.0, "Q"=0.0, "Norm  Ampl"=0.0, "bg (V)"=0.0+0.0i, "4corners"={"z (-pi/2)"=0.0+0.0i, "z(inf)"=0.0+0.0i, "z (pi/2)"=0.0+0.0i, "z center"=0.0+0.0i, "z(0)"=0.0+0.0i, "radius"=0.0}}, "timestamp(min)"=2094.2666666656733, "timestamp"=timestamp(3493853477 s since 1904-01-01), "Magn Field(T)"=0.0}, {"temperature"=14.732, "lorentzian"={"A (VHz)"=0.0, "f (Hz)"=0.0, "G (Hz)"=0.0, "phi(rad)"=0.0, "Q"=0.0, "Norm  Ampl"=0.0, "bg (V)"=0.0+0.0i, "4corners"={"z (-pi/2)"=0.0+0.0i, "z(inf)"=0.0+0.0i, "z (pi/2)"=0.0+0.0i, "z center"=0.0+0.0i, "z(0)"=0.0+0.0i, "radius"=0.0}}, "timestamp(min)"=2095.583333335817, "timestamp"=timestamp(3493853556 s since 1904-01-01), "Magn Field(T)"=0.0}, {"temperature"=14.724, "lorentzian"={"A (VHz)"=0.0, "f (Hz)"=0.0, "G (Hz)"=0.0, "phi(rad)"=0.0, "Q"=0.0, "Norm  Ampl"=0.0, "bg (V)"=0.0+0.0i, "4corners"={"z (-pi/2)"=0.0+0.0i, "z(inf)"=0.0+0.0i, "z (pi/2)"=0.0+0.0i, "z center"=0.0+0.0i, "z(0)"=0.0+0.0i, "radius"=0.0}}, "timestamp(min)"=2096.916666664183, "timestamp"=timestamp(3493853636 s since 1904-01-01), "Magn Field(T)"=0.0}, {"temperature"=14.722, "lorentzian"={"A (VHz)"=0.0, "f (Hz)"=0.0, "G (Hz)"=0.0, "phi(rad)"=0.0, "Q"=0.0, "Norm  Ampl"=0.0, "bg (V)"=0.0+0.0i, "4corners"={"z (-pi/2)"=0.0+0.0i, "z(inf)"=0.0+0.0i, "z (pi/2)"=0.0+0.0i, "z center"=0.0+0.0i, "z(0)"=0.0+0.0i, "radius"=0.0}}, "timestamp(min)"=2098.2333333343267, "timestamp"=timestamp(3493853715 s since 1904-01-01), "Magn Field(T)"=0.0}, {"temperature"=14.72, "lorentzian"={"A (VHz)"=0.0, "f (Hz)"=0.0, "G (Hz)"=0.0, "phi(rad)"=0.0, "Q"=0.0, "Norm  Ampl"=0.0, "bg (V)"=0.0+0.0i, "4corners"={"z (-pi/2)"=0.0+0.0i, "z(inf)"=0.0+0.0i, "z (pi/2)"=0.0+0.0i, "z center"=0.0+0.0i, "z(0)"=0.0+0.0i, "radius"=0.0}}, "timestamp(min)"=2099.5666666701436, "timestamp"=timestamp(3493853795 s since 1904-01-01), "Magn Field(T)"=0.0}, {"temperature"=14.716, "lorentzian"={"A (VHz)"=0.0, "f (Hz)"=0.0, "G (Hz)"=0.0, "phi(rad)"=0.0, "Q"=0.0, "Norm  Ampl"=0.0, "bg (V)"=0.0+0.0i, "4corners"={"z (-pi/2)"=0.0+0.0i, "z(inf)"=0.0+0.0i, "z (pi/2)"=0.0+0.0i, "z center"=0.0+0.0i, "z(0)"=0.0+0.0i, "radius"=0.0}}, "timestamp(min)"=2100.8833333328366, "timestamp"=timestamp(3493853874 s since 1904-01-01), "Magn Field(T)"=0.0}, {"temperature"=14.713, "lorentzian"={"A (VHz)"=0.0, "f (Hz)"=0.0, "G (Hz)"=0.0, "phi(rad)"=0.0, "Q"=0.0, "Norm  Ampl"=0.0, "bg (V)"=0.0+0.0i, "4corners"={"z (-pi/2)"=0.0+0.0i, "z(inf)"=0.0+0.0i, "z (pi/2)"=0.0+0.0i, "z center"=0.0+0.0i, "z(0)"=0.0+0.0i, "radius"=0.0}}, "timestamp(min)"=2102.2000000029802, "timestamp"=timestamp(3493853953 s since 1904-01-01), "Magn Field(T)"=0.0}, {"temperature"=14.71, "lorentzian"={"A (VHz)"=0.0, "f (Hz)"=0.0, "G (Hz)"=0.0, "phi(rad)"=0.0, "Q"=0.0, "Norm  Ampl"=0.0, "bg (V)"=0.0+0.0i, "4corners"={"z (-pi/2)"=0.0+0.0i, "z(inf)"=0.0+0.0i, "z (pi/2)"=0.0+0.0i, "z center"=0.0+0.0i, "z(0)"=0.0+0.0i, "radius"=0.0}}, "timestamp(min)"=2103.5333333313465, "timestamp"=timestamp(3493854033 s since 1904-01-01), "Magn Field(T)"=0.0}, {"temperature"=14.704, "lorentzian"={"A (VHz)"=0.0, "f (Hz)"=0.0, "G (Hz)"=0.0, "phi(rad)"=0.0, "Q"=0.0, "Norm  Ampl"=0.0, "bg (V)"=0.0+0.0i, "4corners"={"z (-pi/2)"=0.0+0.0i, "z(inf)"=0.0+0.0i, "z (pi/2)"=0.0+0.0i, "z center"=0.0+0.0i, "z(0)"=0.0+0.0i, "radius"=0.0}}, "timestamp(min)"=2104.85000000149, "timestamp"=timestamp(3493854112 s since 1904-01-01), "Magn Field(T)"=0.0}, {"temperature"=14.705, "lorentzian"={"A (VHz)"=0.0, "f (Hz)"=0.0, "G (Hz)"=0.0, "phi(rad)"=0.0, "Q"=0.0, "Norm  Ampl"=0.0, "bg (V)"=0.0+0.0i, "4corners"={"z (-pi/2)"=0.0+0.0i, "z(inf)"=0.0+0.0i, "z (pi/2)"=0.0+0.0i, "z center"=0.0+0.0i, "z(0)"=0.0+0.0i, "radius"=0.0}}, "timestamp(min)"=2106.166666664183, "timestamp"=timestamp(3493854191 s since 1904-01-01), "Magn Field(T)"=0.0}, {"temperature"=14.703, "lorentzian"={"A (VHz)"=0.0, "f (Hz)"=0.0, "G (Hz)"=0.0, "phi(rad)"=0.0, "Q"=0.0, "Norm  Ampl"=0.0, "bg (V)"=0.0+0.0i, "4corners"={"z (-pi/2)"=0.0+0.0i, "z(inf)"=0.0+0.0i, "z (pi/2)"=0.0+0.0i, "z center"=0.0+0.0i, "z(0)"=0.0+0.0i, "radius"=0.0}}, "timestamp(min)"=2107.5, "timestamp"=timestamp(3493854271 s since 1904-01-01), "Magn Field(T)"=0.0}, {"temperature"=14.7, "lorentzian"={"A (VHz)"=0.0, "f (Hz)"=0.0, "G (Hz)"=0.0, "phi(rad)"=0.0, "Q"=0.0, "Norm  Ampl"=0.0, "bg (V)"=0.0+0.0i, "4corners"={"z (-pi/2)"=0.0+0.0i, "z(inf)"=0.0+0.0i, "z (pi/2)"=0.0+0.0i, "z center"=0.0+0.0i, "z(0)"=0.0+0.0i, "radius"=0.0}}, "timestamp(min)"=2108.8166666701436, "timestamp"=timestamp(3493854350 s since 1904-01-01), "Magn Field(T)"=0.0}, {"temperature"=14.697, "lorentzian"={"A (VHz)"=0.0, "f (Hz)"=0.0, "G (Hz)"=0.0, "phi(rad)"=0.0, "Q"=0.0, "Norm  Ampl"=0.0, "bg (V)"=0.0+0.0i, "4corners"={"z (-pi/2)"=0.0+0.0i, "z(inf)"=0.0+0.0i, "z (pi/2)"=0.0+0.0i, "z center"=0.0+0.0i, "z(0)"=0.0+0.0i, "radius"=0.0}}, "timestamp(min)"=2110.14999999851, "timestamp"=timestamp(3493854430 s since 1904-01-01), "Magn Field(T)"=0.0}, {"temperature"=14.688, "lorentzian"={"A (VHz)"=0.0, "f (Hz)"=0.0, "G (Hz)"=0.0, "phi(rad)"=0.0, "Q"=0.0, "Norm  Ampl"=0.0, "bg (V)"=0.0+0.0i, "4corners"={"z (-pi/2)"=0.0+0.0i, "z(inf)"=0.0+0.0i, "z (pi/2)"=0.0+0.0i, "z center"=0.0+0.0i, "z(0)"=0.0+0.0i, "radius"=0.0}}, "timestamp(min)"=2111.4666666686535, "timestamp"=timestamp(3493854509 s since 1904-01-01), "Magn Field(T)"=0.0}, {"temperature"=14.695, "lorentzian"={"A (VHz)"=0.0, "f (Hz)"=0.0, "G (Hz)"=0.0, "phi(rad)"=0.0, "Q"=0.0, "Norm  Ampl"=0.0, "bg (V)"=0.0+0.0i, "4corners"={"z (-pi/2)"=0.0+0.0i, "z(inf)"=0.0+0.0i, "z (pi/2)"=0.0+0.0i, "z center"=0.0+0.0i, "z(0)"=0.0+0.0i, "radius"=0.0}}, "timestamp(min)"=2112.7833333313465, "timestamp"=timestamp(3493854588 s since 1904-01-01), "Magn Field(T)"=0.0}, {"temperature"=14.696, "lorentzian"={"A (VHz)"=0.0, "f (Hz)"=0.0, "G (Hz)"=0.0, "phi(rad)"=0.0, "Q"=0.0, "Norm  Ampl"=0.0, "bg (V)"=0.0+0.0i, "4corners"={"z (-pi/2)"=0.0+0.0i, "z(inf)"=0.0+0.0i, "z (pi/2)"=0.0+0.0i, "z center"=0.0+0.0i, "z(0)"=0.0+0.0i, "radius"=0.0}}, "timestamp(min)"=2114.1166666671634, "timestamp"=timestamp(3493854668 s since 1904-01-01), "Magn Field(T)"=0.0}, {"temperature"=14.691, "lorentzian"={"A (VHz)"=0.0, "f (Hz)"=0.0, "G (Hz)"=0.0, "phi(rad)"=0.0, "Q"=0.0, "Norm  Ampl"=0.0, "bg (V)"=0.0+0.0i, "4corners"={"z (-pi/2)"=0.0+0.0i, "z(inf)"=0.0+0.0i, "z (pi/2)"=0.0+0.0i, "z center"=0.0+0.0i, "z(0)"=0.0+0.0i, "radius"=0.0}}, "timestamp(min)"=2115.433333337307, "timestamp"=timestamp(3493854747 s since 1904-01-01), "Magn Field(T)"=0.0}, {"temperature"=14.69, "lorentzian"={"A (VHz)"=0.0, "f (Hz)"=0.0, "G (Hz)"=0.0, "phi(rad)"=0.0, "Q"=0.0, "Norm  Ampl"=0.0, "bg (V)"=0.0+0.0i, "4corners"={"z (-pi/2)"=0.0+0.0i, "z(inf)"=0.0+0.0i, "z (pi/2)"=0.0+0.0i, "z center"=0.0+0.0i, "z(0)"=0.0+0.0i, "radius"=0.0}}, "timestamp(min)"=2116.75, "timestamp"=timestamp(3493854826 s since 1904-01-01), "Magn Field(T)"=0.0}, {"temperature"=14.69, "lorentzian"={"A (VHz)"=0.0, "f (Hz)"=0.0, "G (Hz)"=0.0, "phi(rad)"=0.0, "Q"=0.0, "Norm  Ampl"=0.0, "bg (V)"=0.0+0.0i, "4corners"={"z (-pi/2)"=0.0+0.0i, "z(inf)"=0.0+0.0i, "z (pi/2)"=0.0+0.0i, "z center"=0.0+0.0i, "z(0)"=0.0+0.0i, "radius"=0.0}}, "timestamp(min)"=2118.083333335817, "timestamp"=timestamp(3493854906 s since 1904-01-01), "Magn Field(T)"=0.0}, {"temperature"=14.686, "lorentzian"={"A (VHz)"=0.0, "f (Hz)"=0.0, "G (Hz)"=0.0, "phi(rad)"=0.0, "Q"=0.0, "Norm  Ampl"=0.0, "bg (V)"=0.0+0.0i, "4corners"={"z (-pi/2)"=0.0+0.0i, "z(inf)"=0.0+0.0i, "z (pi/2)"=0.0+0.0i, "z center"=0.0+0.0i, "z(0)"=0.0+0.0i, "radius"=0.0}}, "timestamp(min)"=2119.39999999851, "timestamp"=timestamp(3493854985 s since 1904-01-01), "Magn Field(T)"=0.0}, {"temperature"=14.682, "lorentzian"={"A (VHz)"=0.0, "f (Hz)"=0.0, "G (Hz)"=0.0, "phi(rad)"=0.0, "Q"=0.0, "Norm  Ampl"=0.0, "bg (V)"=0.0+0.0i, "4corners"={"z (-pi/2)"=0.0+0.0i, "z(inf)"=0.0+0.0i, "z (pi/2)"=0.0+0.0i, "z center"=0.0+0.0i, "z(0)"=0.0+0.0i, "radius"=0.0}}, "timestamp(min)"=2120.7333333343267, "timestamp"=timestamp(3493855065 s since 1904-01-01), "Magn Field(T)"=0.0}, {"temperature"=14.684, "lorentzian"={"A (VHz)"=0.0, "f (Hz)"=0.0, "G (Hz)"=0.0, "phi(rad)"=0.0, "Q"=0.0, "Norm  Ampl"=0.0, "bg (V)"=0.0+0.0i, "4corners"={"z (-pi/2)"=0.0+0.0i, "z(inf)"=0.0+0.0i, "z (pi/2)"=0.0+0.0i, "z center"=0.0+0.0i, "z(0)"=0.0+0.0i, "radius"=0.0}}, "timestamp(min)"=2122.0500000044703, "timestamp"=timestamp(3493855144 s since 1904-01-01), "Magn Field(T)"=0.0}, {"temperature"=14.679, "lorentzian"={"A (VHz)"=0.0, "f (Hz)"=0.0, "G (Hz)"=0.0, "phi(rad)"=0.0, "Q"=0.0, "Norm  Ampl"=0.0, "bg (V)"=0.0+0.0i, "4corners"={"z (-pi/2)"=0.0+0.0i, "z(inf)"=0.0+0.0i, "z (pi/2)"=0.0+0.0i, "z center"=0.0+0.0i, "z(0)"=0.0+0.0i, "radius"=0.0}}, "timestamp(min)"=2123.3666666671634, "timestamp"=timestamp(3493855223 s since 1904-01-01), "Magn Field(T)"=0.0}, {"temperature"=14.677, "lorentzian"={"A (VHz)"=0.0, "f (Hz)"=0.0, "G (Hz)"=0.0, "phi(rad)"=0.0, "Q"=0.0, "Norm  Ampl"=0.0, "bg (V)"=0.0+0.0i, "4corners"={"z (-pi/2)"=0.0+0.0i, "z(inf)"=0.0+0.0i, "z (pi/2)"=0.0+0.0i, "z center"=0.0+0.0i, "z(0)"=0.0+0.0i, "radius"=0.0}}, "timestamp(min)"=2124.7000000029802, "timestamp"=timestamp(3493855303 s since 1904-01-01), "Magn Field(T)"=0.0}, {"temperature"=14.676, "lorentzian"={"A (VHz)"=0.0, "f (Hz)"=0.0, "G (Hz)"=0.0, "phi(rad)"=0.0, "Q"=0.0, "Norm  Ampl"=0.0, "bg (V)"=0.0+0.0i, "4corners"={"z (-pi/2)"=0.0+0.0i, "z(inf)"=0.0+0.0i, "z (pi/2)"=0.0+0.0i, "z center"=0.0+0.0i, "z(0)"=0.0+0.0i, "radius"=0.0}}, "timestamp(min)"=2126.0166666656733, "timestamp"=timestamp(3493855382 s since 1904-01-01), "Magn Field(T)"=0.0}, {"temperature"=14.671, "lorentzian"={"A (VHz)"=0.0, "f (Hz)"=0.0, "G (Hz)"=0.0, "phi(rad)"=0.0, "Q"=0.0, "Norm  Ampl"=0.0, "bg (V)"=0.0+0.0i, "4corners"={"z (-pi/2)"=0.0+0.0i, "z(inf)"=0.0+0.0i, "z (pi/2)"=0.0+0.0i, "z center"=0.0+0.0i, "z(0)"=0.0+0.0i, "radius"=0.0}}, "timestamp(min)"=2127.35000000149, "timestamp"=timestamp(3493855462 s since 1904-01-01), "Magn Field(T)"=0.0}, {"temperature"=14.665, "lorentzian"={"A (VHz)"=0.0, "f (Hz)"=0.0, "G (Hz)"=0.0, "phi(rad)"=0.0, "Q"=0.0, "Norm  Ampl"=0.0, "bg (V)"=0.0+0.0i, "4corners"={"z (-pi/2)"=0.0+0.0i, "z(inf)"=0.0+0.0i, "z (pi/2)"=0.0+0.0i, "z center"=0.0+0.0i, "z(0)"=0.0+0.0i, "radius"=0.0}}, "timestamp(min)"=2128.666666664183, "timestamp"=timestamp(3493855541 s since 1904-01-01), "Magn Field(T)"=0.0}, {"temperature"=14.666, "lorentzian"={"A (VHz)"=0.0, "f (Hz)"=0.0, "G (Hz)"=0.0, "phi(rad)"=0.0, "Q"=0.0, "Norm  Ampl"=0.0, "bg (V)"=0.0+0.0i, "4corners"={"z (-pi/2)"=0.0+0.0i, "z(inf)"=0.0+0.0i, "z (pi/2)"=0.0+0.0i, "z center"=0.0+0.0i, "z(0)"=0.0+0.0i, "radius"=0.0}}, "timestamp(min)"=2129.9833333343267, "timestamp"=timestamp(3493855620 s since 1904-01-01), "Magn Field(T)"=0.0}, {"temperature"=14.661, "lorentzian"={"A (VHz)"=0.0, "f (Hz)"=0.0, "G (Hz)"=0.0, "phi(rad)"=0.0, "Q"=0.0, "Norm  Ampl"=0.0, "bg (V)"=0.0+0.0i, "4corners"={"z (-pi/2)"=0.0+0.0i, "z(inf)"=0.0+0.0i, "z (pi/2)"=0.0+0.0i, "z center"=0.0+0.0i, "z(0)"=0.0+0.0i, "radius"=0.0}}, "timestamp(min)"=2131.3166666701436, "timestamp"=timestamp(3493855700 s since 1904-01-01), "Magn Field(T)"=0.0}, {"temperature"=14.654, "lorentzian"={"A (VHz)"=0.0, "f (Hz)"=0.0, "G (Hz)"=0.0, "phi(rad)"=0.0, "Q"=0.0, "Norm  Ampl"=0.0, "bg (V)"=0.0+0.0i, "4corners"={"z (-pi/2)"=0.0+0.0i, "z(inf)"=0.0+0.0i, "z (pi/2)"=0.0+0.0i, "z center"=0.0+0.0i, "z(0)"=0.0+0.0i, "radius"=0.0}}, "timestamp(min)"=2132.6333333328366, "timestamp"=timestamp(3493855779 s since 1904-01-01), "Magn Field(T)"=0.0}, {"temperature"=14.654, "lorentzian"={"A (VHz)"=0.0, "f (Hz)"=0.0, "G (Hz)"=0.0, "phi(rad)"=0.0, "Q"=0.0, "Norm  Ampl"=0.0, "bg (V)"=0.0+0.0i, "4corners"={"z (-pi/2)"=0.0+0.0i, "z(inf)"=0.0+0.0i, "z (pi/2)"=0.0+0.0i, "z center"=0.0+0.0i, "z(0)"=0.0+0.0i, "radius"=0.0}}, "timestamp(min)"=2133.9500000029802, "timestamp"=timestamp(3493855858 s since 1904-01-01), "Magn Field(T)"=0.0}, {"temperature"=14.648, "lorentzian"={"A (VHz)"=0.0, "f (Hz)"=0.0, "G (Hz)"=0.0, "phi(rad)"=0.0, "Q"=0.0, "Norm  Ampl"=0.0, "bg (V)"=0.0+0.0i, "4corners"={"z (-pi/2)"=0.0+0.0i, "z(inf)"=0.0+0.0i, "z (pi/2)"=0.0+0.0i, "z center"=0.0+0.0i, "z(0)"=0.0+0.0i, "radius"=0.0}}, "timestamp(min)"=2135.2833333313465, "timestamp"=timestamp(3493855938 s since 1904-01-01), "Magn Field(T)"=0.0}, {"temperature"=14.653, "lorentzian"={"A (VHz)"=0.0, "f (Hz)"=0.0, "G (Hz)"=0.0, "phi(rad)"=0.0, "Q"=0.0, "Norm  Ampl"=0.0, "bg (V)"=0.0+0.0i, "4corners"={"z (-pi/2)"=0.0+0.0i, "z(inf)"=0.0+0.0i, "z (pi/2)"=0.0+0.0i, "z center"=0.0+0.0i, "z(0)"=0.0+0.0i, "radius"=0.0}}, "timestamp(min)"=2136.60000000149, "timestamp"=timestamp(3493856017 s since 1904-01-01), "Magn Field(T)"=0.0}, {"temperature"=14.656, "lorentzian"={"A (VHz)"=0.0, "f (Hz)"=0.0, "G (Hz)"=0.0, "phi(rad)"=0.0, "Q"=0.0, "Norm  Ampl"=0.0, "bg (V)"=0.0+0.0i, "4corners"={"z (-pi/2)"=0.0+0.0i, "z(inf)"=0.0+0.0i, "z (pi/2)"=0.0+0.0i, "z center"=0.0+0.0i, "z(0)"=0.0+0.0i, "radius"=0.0}}, "timestamp(min)"=2137.933333337307, "timestamp"=timestamp(3493856097 s since 1904-01-01), "Magn Field(T)"=0.0}, {"temperature"=14.654, "lorentzian"={"A (VHz)"=0.0, "f (Hz)"=0.0, "G (Hz)"=0.0, "phi(rad)"=0.0, "Q"=0.0, "Norm  Ampl"=0.0, "bg (V)"=0.0+0.0i, "4corners"={"z (-pi/2)"=0.0+0.0i, "z(inf)"=0.0+0.0i, "z (pi/2)"=0.0+0.0i, "z center"=0.0+0.0i, "z(0)"=0.0+0.0i, "radius"=0.0}}, "timestamp(min)"=2139.25, "timestamp"=timestamp(3493856176 s since 1904-01-01), "Magn Field(T)"=0.0}, {"temperature"=14.646, "lorentzian"={"A (VHz)"=0.0, "f (Hz)"=0.0, "G (Hz)"=0.0, "phi(rad)"=0.0, "Q"=0.0, "Norm  Ampl"=0.0, "bg (V)"=0.0+0.0i, "4corners"={"z (-pi/2)"=0.0+0.0i, "z(inf)"=0.0+0.0i, "z (pi/2)"=0.0+0.0i, "z center"=0.0+0.0i, "z(0)"=0.0+0.0i, "radius"=0.0}}, "timestamp(min)"=2140.5666666701436, "timestamp"=timestamp(3493856255 s since 1904-01-01), "Magn Field(T)"=0.0}, {"temperature"=14.643, "lorentzian"={"A (VHz)"=0.0, "f (Hz)"=0.0, "G (Hz)"=0.0, "phi(rad)"=0.0, "Q"=0.0, "Norm  Ampl"=0.0, "bg (V)"=0.0+0.0i, "4corners"={"z (-pi/2)"=0.0+0.0i, "z(inf)"=0.0+0.0i, "z (pi/2)"=0.0+0.0i, "z center"=0.0+0.0i, "z(0)"=0.0+0.0i, "radius"=0.0}}, "timestamp(min)"=2141.89999999851, "timestamp"=timestamp(3493856335 s since 1904-01-01), "Magn Field(T)"=0.0}, {"temperature"=14.643, "lorentzian"={"A (VHz)"=0.0, "f (Hz)"=0.0, "G (Hz)"=0.0, "phi(rad)"=0.0, "Q"=0.0, "Norm  Ampl"=0.0, "bg (V)"=0.0+0.0i, "4corners"={"z (-pi/2)"=0.0+0.0i, "z(inf)"=0.0+0.0i, "z (pi/2)"=0.0+0.0i, "z center"=0.0+0.0i, "z(0)"=0.0+0.0i, "radius"=0.0}}, "timestamp(min)"=2143.2166666686535, "timestamp"=timestamp(3493856414 s since 1904-01-01), "Magn Field(T)"=0.0}, {"temperature"=14.638, "lorentzian"={"A (VHz)"=0.0, "f (Hz)"=0.0, "G (Hz)"=0.0, "phi(rad)"=0.0, "Q"=0.0, "Norm  Ampl"=0.0, "bg (V)"=0.0+0.0i, "4corners"={"z (-pi/2)"=0.0+0.0i, "z(inf)"=0.0+0.0i, "z (pi/2)"=0.0+0.0i, "z center"=0.0+0.0i, "z(0)"=0.0+0.0i, "radius"=0.0}}, "timestamp(min)"=2144.5333333313465, "timestamp"=timestamp(3493856493 s since 1904-01-01), "Magn Field(T)"=0.0}, {"temperature"=14.634, "lorentzian"={"A (VHz)"=0.0, "f (Hz)"=0.0, "G (Hz)"=0.0, "phi(rad)"=0.0, "Q"=0.0, "Norm  Ampl"=0.0, "bg (V)"=0.0+0.0i, "4corners"={"z (-pi/2)"=0.0+0.0i, "z(inf)"=0.0+0.0i, "z (pi/2)"=0.0+0.0i, "z center"=0.0+0.0i, "z(0)"=0.0+0.0i, "radius"=0.0}}, "timestamp(min)"=2145.8666666671634, 
